vi "getAllFrames.vi"(8 "error in (no error)":errorcluster, 10 "1st occurrence":refnum<k4>, 11 "IMAQ Session In":refnum<k11>) -> (0 "error out":errorcluster, 1 "Updated camera":T2, 2 "Finished Acquisition":bool, 3 "Encountered Trigger":bool)   [LabVIEW 2017]
uses:
  <vilib>/vision/Image Controls.llb/IMAQ Image.ctl
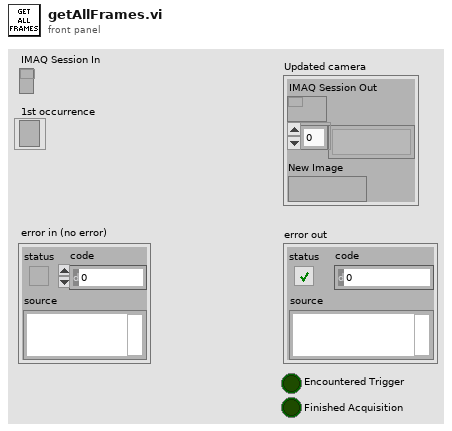
[diagram p1: front panel]
types:
  T1 = typedef "IMAQ Image.ctl" = refnum<image>
  T2 = cluster{"IMAQ Session Out":refnum<k11>, T1[], "New Image":T1}
  T3 = cluster{"IMAQ Session Out":refnum<k11>, "Images Out":T1[], "New Image":T1}
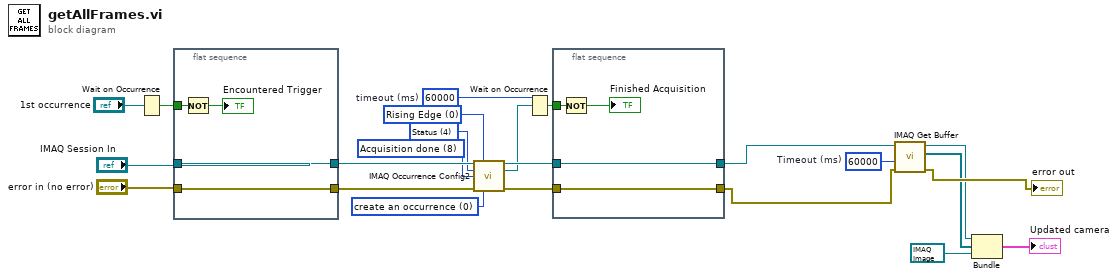
[diagram p0: block diagram]
diagram:
  w6 = 60000  # Timeout (ms)
  w13 = 60000  # timeout (ms)
  w14 = u16 0 items=["create an occurrence", "clear all occurrences"] ("create/clear")
  w15 = u32 8 items=["Acquisition in progress"=15, "Acquisition done"=8, "Frame start"=9, "Frame done"=10, "Buffer Complete"=11] ("Status Signal")
  w16 = u32 4 items=["External", "RTSI ", "ISO In", "ISO Out", "Status"] ("Signal Type")
  w17 = u32 0 items=["Rising Edge", "Falling Edge"] ("Signal polarity")
  n1 = Wait on Occurrence(2:"1st occurrence") -> (0:w12:bool)  [unwired: 2 in]
  n2 = flat-sequence {
    tunnel: w12 -> [w27]
    tunnel: "error in (no error)" -> [w26]
    tunnel: [w24] -> w18
    tunnel: [w26] -> w19
    tunnel: "IMAQ Session In" -> [w24]
    frame #0 {
      n3 = Not(x=w27) -> (.not. x?=→"Encountered Trigger":bool)
    }
  }
  n4 = call <vilib>:"IMAQ Occurrence Config2.vi"("IMAQ Session In"=w18, "Signal polarity"=w17, "Signal Type"=w16, "Status Signal"=w15, "error in (no error)"=w19, "create/clear"=w14) -> ("IMAQ Session Out"=w22:refnum<k11>, "occurrence"=w20:refnum<k4>, "error out"=w23:errorcluster)  [unwired: 7 in]
  n5 = Wait on Occurrence(2:w20, 3:w13) -> (0:w21:bool)  [unwired: 1 in]
  n6 = flat-sequence {
    tunnel: w21 -> [w29]
    tunnel: w23 -> [w30]
    tunnel: w22 -> [w31]
    tunnel: [w31] -> w5
    tunnel: [w30] -> w4
    frame #0 {
      n7 = Not(x=w29) -> (.not. x?=→"Finished Acquisition":bool)
    }
  }
  n8 = call <vilib>:"IMAQ Get Buffer.vi"("error in (no error)"=w4, "Timeout (ms)"=w6, "IMAQ Session In"=w5) -> ("error out"=→"error out":errorcluster, "Images Out"=w1:T1[], "IMAQ Session Out"=w2:refnum<k11>)  [unwired: 1 in, 5 out]
  n9 = Bundle("IMAQ Session Out"=w2, "Images Out"=w1, "New Image"=T1 refnum) -> (→"Updated camera":T3)  [unwired: 1 in]
